vi "Calcula tração com temperatura alvo.vi"(4 "A1 (m)":dbl=500.0, 5 "t2-t1 (°C)":dbl=35.0, 6 "To1 (N)":dbl=18350.0, 7 "Alfa t (1/°C)":dbl=2.09e-05, 8 "E (Pa)":dbl=65500000000.0, 9 "S (m²)":dbl=0.0005168, 10 "p (N/m)":dbl=18.35, 11 "Ao (m)":dbl=500.0) -> (2 "To2 Real  (N)":dbl=17749.49999999993 format="%.3f")   [LabVIEW 2020]
doc: "Calculo da tração com temperatura diferente da EDS"
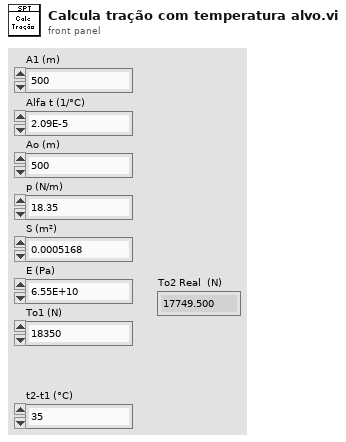
[diagram p1: front panel]
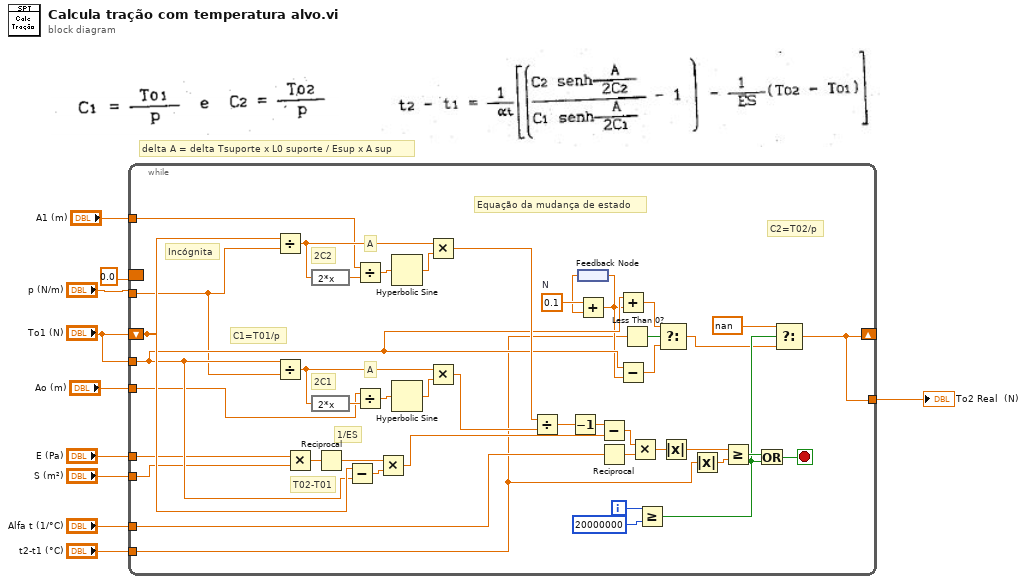
[diagram p0: block diagram]
diagram:
  # "delta A = delta Tsuporte x L0 suporte / Esup x A sup"
  n1 = while {
    shift-right: [w11] -> _
    shift-left: "To1 (N)" -> [w33]
    tunnel: "To1 (N)" -> [w29]
    border: 0.0 -> [_]
    tunnel: "E (Pa)" -> [w25]
    tunnel: "S (m²)" -> [w24]
    tunnel: "t2-t1 (°C)" -> [w19]
    tunnel: "Alfa t (1/°C)" -> [w23]
    tunnel: "p (N/m)" -> [w22]
    tunnel: [w11] -> w3
    tunnel: "Ao (m)" -> [w21]
    tunnel: "A1 (m)" -> [w20]
    i -> [w18]
    stop <- w16 stop-if-true
    w35 = 0.1  # N
    # "Equação da mudança de estado"
    # "Incógnita"
    # "T02-T01"
    # "1/ES"
    # "C1=T01/p"
    # "A"
    # "2C1"
    # "C2=T02/p"
    # "A"
    # "2C2"
    n2 = Divide(x=w33, y=w22) -> (x/y=w51:dbl)
    n3 = Divide(x=w29, y=w22) -> (x/y=w50:dbl)
    n4 = Multiply(x=w25, y=w24) -> (x*y=w42:dbl)
    n5 = expression code="2*x"(w51) -> (w52:dbl)
    n6 = expression code="2*x"(w50) -> (w49:dbl)
    n7 = Reciprocal(x=w42) -> (1/x=w41:dbl)
    n8 = Subtract(x=w33, y=w29) -> (x-y=w40:dbl)
    n9 = Divide(x=w20, y=w52) -> (x/y=w54:dbl)
    n10 = Divide(x=w21, y=w49) -> (x/y=w47:dbl)
    n11 = Multiply(x=w41, y=w40) -> (x*y=w39:dbl)
    n12 = Hyperbolic Sine(1:w54) -> (0:w53:dbl)
    n13 = Hyperbolic Sine(1:w47) -> (0:w48:dbl)
    n14 = Multiply(x=w51, y=w53) -> (x*y=w46:dbl)
    n15 = Multiply(x=w50, y=w48) -> (x*y=w45:dbl)
    n16 = Divide(x=w46, y=w45) -> (x/y=w44:dbl)
    n17 = Decrement(x=w44) -> (x-1=w43:dbl)
    n18 = feedback #1() -> (w34:dbl)
    n19 = Add(x=w35, y=w34) -> (x+y=w28:dbl)
    n20 = feedback-in #1(w28) -> ()
    n21 = Subtract(x=w43, y=w39) -> (x-y=w38:dbl)
    n22 = Reciprocal(x=w23) -> (1/x=w37:dbl)
    n23 = Add(x=w29, y=w28) -> (x+y=w30:dbl)
    n24 = Subtract(x=w29, y=w28) -> (x-y=w31:dbl)
    n25 = Less Than 0?(x=w19) -> (x < 0?=w32:bool)
    n26 = Multiply(x=w38, y=w37) -> (x*y=w36:dbl)
    n27 = Greater Or Equal?(x=w18, y=20000000) -> (x >= y?=w14:bool)
    n28 = Select(t=w30, s=w32, f=w31) -> (s? t:f=w12:dbl)
    n29 = Absolute Value(x=w36) -> (abs(x)=w26:dbl)
    n30 = Absolute Value(x=w19) -> (abs(x)=w27:dbl)
    n31 = Greater Or Equal?(x=w26, y=w27) -> (x >= y?=w15:bool)
    n32 = Or(x=w15, y=w14) -> (x .or. y?=w16:bool)
    n33 = Select(t=nan, s=w14, f=w12) -> (s? t:f=w11:dbl)
  }
  "To2 Real  (N)" <- w3
